vi "index.vi"(10 "Array":i32[](array[numeric])) -> (2 "x/y":dbl[](array[numeric]))   [LabVIEW 2013]
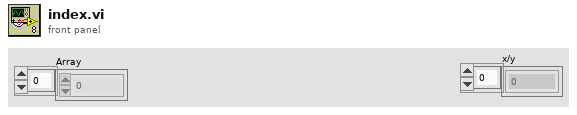
[diagram p1: front panel]
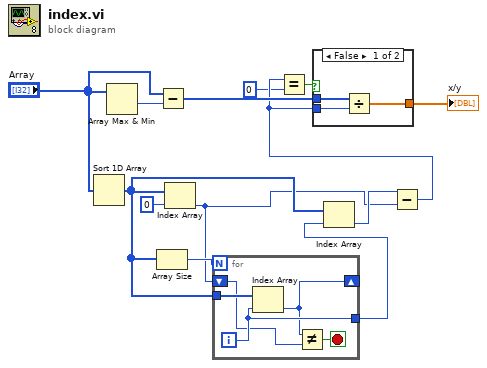
[diagram p0: block diagram]
diagram:
  n1 = Sort 1D Array(array="Array") -> (sorted array=w4:i32[])
  n2 = Array Max & Min(array="Array") -> (min value=w13:i32)  [unwired: 3 out]
  n3 = Array Size(array=w4) -> (size(s)=w6:i32)
  n4 = Subtract(x="Array", y=w13) -> (x-y=w11:i32[])
  n5 = Index Array(array=w4, index=0) -> (element=w1:i32)
  n6 = for {
    N: w6 -> [_]
    tunnel: w4 -> [w18]
    tunnel: [w17] -> w3
    shift-right: [w15] -> _
    shift-left: w1 -> [w14]
    i -> [w17]
    stop <- w16 stop-if-true
    n7 = Index Array(array=w18, index=w17) -> (element=w15:i32)
    n8 = Not Equal?(x=w15, y=w14) -> (x != y?=w16:bool)
  }
  n9 = Index Array(array=w4, index=w3) -> (element=w2:i32)
  n10 = Subtract(x=w2, y=w1) -> (x-y=w8:i32)
  n11 = Equal?(x=w8, y=0) -> (x = y?=w9:bool)
  n12 = case shown="False" w9 {
    tunnel: w8 -> [w21 _]
    tunnel: w11 -> [w20 w22]
    tunnel: [w19 w22] -> w10
    frame False {
      n13 = Divide(x=w20, y=w21) -> (x/y=w19:dbl[])
    }
    frame True {
    }
  }
  "x/y" <- w10
